vi "Config VI.vi"(8 "error in (no error)":errorcluster, 11 "Plugin in":refnum<class "Plugin.lvclass">) -> (0 "error out":errorcluster, 3 "Plugin out":refnum<class "Plugin.lvclass">)   [LabVIEW 2015, in "ProjectLoader.lvclass"]
uses:
  ProjectLoader.lvclass
  Core/Plugin.lvclass
  Core/Plugin/Plugin Config UI State.ctl
  JsonReportPlugin.lvclass
panel:
  in  "Enable":bool
  in  "Project File":path
  in  "Load Type":enum32{"Manually", "Automatic"}(radio)
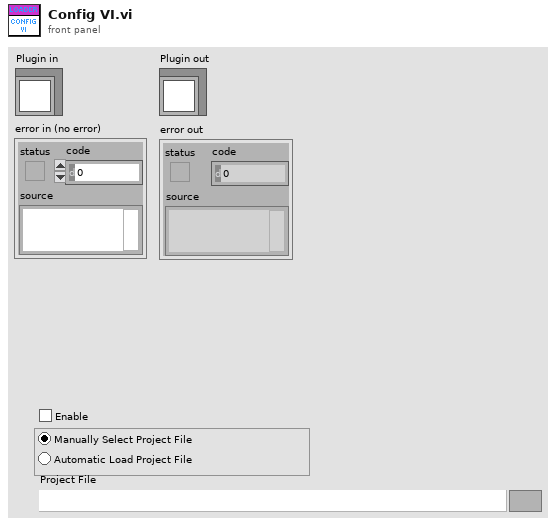
[diagram p1: front panel]
types:
  T1 = typedef "Plugin.lvclass/Plugin Config UI State.ctl" = enum16{"UI_LOOP", "INIT", "END"}
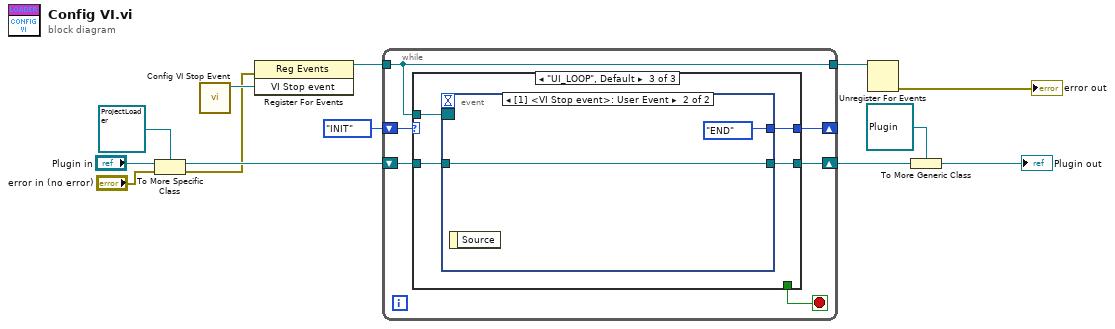
[diagram p0: block diagram]
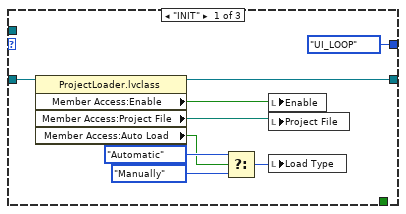
[diagram p2: hidden frame]
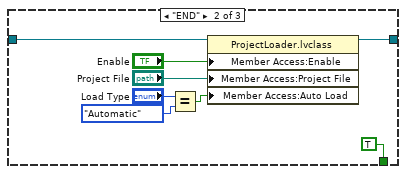
[diagram p3: hidden frame]
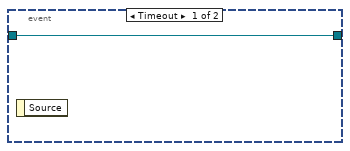
[diagram p4: hidden frame]
diagram:
  n1 = To More Specific Class(target class=refnum<class "ProjectLoader.lvclass"> refnum ("ProjectLoader.lvclass"), reference="Plugin in", error in="error in (no error)") -> (specific class reference=w3:refnum<class "ProjectLoader.lvclass">, error out=w2:errorcluster)
  n2 = call "Config VI Stop Event.vi"() -> ("VI Stop event"=w13:refnum<user-event>)  [unwired: 11 in]
  n3 = register-events(error in=w2, w13) -> (reference out=w12:refnum<event-registration>)  [unwired: 1 in, 1 out]
  n4 = while {
    tunnel: w12 -> [w18]
    tunnel: [w18] -> w11
    shift-right: [w16] -> _
    shift-left: Plugin_Config_UI_State."INIT" ("State") -> [w17]
    shift-right: [w14] -> w1
    shift-left: w3 -> [w15]
    stop <- w19 stop-if-true
    n5 = case shown="\"UI_LOOP\", Default" w17 {
      tunnel: [_ TRUE _] -> w19
      tunnel: w18 -> [_ _ w40]
      tunnel: [Plugin_Config_UI_State."UI_LOOP" ("State") _ w39] -> w16
      tunnel: w15 -> [w27 w35 w38]
      tunnel: [w24 w34 w37] -> w14
      frame "INIT" {
        n6 = property class="ProjectLoader.lvclass"(reference=w27) -> (reference out=w24:refnum<class "ProjectLoader.lvclass">, "Member Access:Enable"=w26:bool, "Member Access:Project File"=w25:path, "Member Access:Auto Load"=w21:bool)  [unwired: 1 in, 1 out]
        n7 = Select(t=enum32{"Manually", "Automatic"}."Automatic" ("Load Type"), s=w21, f=enum32{"Manually", "Automatic"}."Manually" ("Load Type")) -> (s? t:f=w20:enum32{"Manually", "Automatic"})
        n8 = local write "Enable"(w26) -> ()
        n9 = local write "Project File"(w25) -> ()
        n10 = local write "Load Type"(w20) -> ()
      }
      frame "END" {
        n11 = Equal?(x="Load Type", y=enum32{"Manually", "Automatic"}."Automatic" ("Load Type")) -> (x = y?=w29:bool)
        n12 = property class="ProjectLoader.lvclass"(reference=w35, "Member Access:Enable"="Enable", "Member Access:Project File"="Project File", "Member Access:Auto Load"=w29) -> (reference out=w34:refnum<class "ProjectLoader.lvclass">)  [unwired: 1 in, 1 out]
      }
      frame "UI_LOOP", Default {
        n13 = event shown="[1] <VI Stop event>: User Event" {
          selector: w40 -> [_ _]
          dyn-events: _ -> [_ _]
          timeout: _ -> [_ _]
          tunnel: [_ Plugin_Config_UI_State."END" ("State")] -> w39
          tunnel: w38 -> [w41 w42]
          tunnel: [w41 w42] -> w37
          event Timeout {
            n14 = event-data() -> ()  [unwired: 1 in, 1 out]
          }
          event User Event {
            n15 = event-data() -> ()  [unwired: 1 in, 1 out]
          }
        }
      }
    }
  }
  n16 = Unregister For Events(event registration refnum=w11) -> (error out=→"error out":errorcluster)  [unwired: 1 in]
  n17 = To More Generic Class(target class=refnum<class "Plugin.lvclass"> refnum ("Plugin out"), reference=w1) -> (generic class reference=→"Plugin out":refnum<class "Plugin.lvclass">)
